vi "Handle LogRec.vi"(8 "error in":errorcluster, 10 "LogRecord":refnum<class "LogRecord.lvclass">, 11 "LokiHandler in":refnum<class "LokiHandler.lvclass">) -> (0 "error out":errorcluster, 3 "LokiHandler out":refnum<class "LokiHandler.lvclass">)   [LabVIEW 2017, in "hse-logger.lvlib" / "LokiHandler.lvclass"]
doc: "Handles the incoming ``LogRecord`` object.\n\nThis method is the implementation of the base-class and does nothing. Use a pre-defined sub-class or implement your own."
uses:
  LokiHandler.lvclass
  LokiHandler.lvclass/LokiHandler.ctl
  LogRecord/LogRecord.lvclass
  <vilib>/httpClient/LabVIEWHTTPClient.lvlib
  <vilib>/httpClient/POSTBuffer.vi
  Formatter/LokiJsonFormatter/LokiJsonFormatter.lvclass
panel:
  # "Connector Pane"
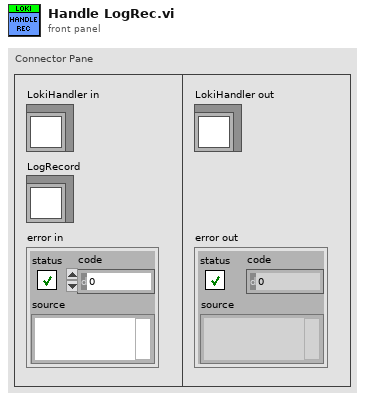
[diagram p1: front panel]
types:
  T1 = typedef "hse-logger.lvlib/LogLevel.ctl" = enum16{"DEBUG", "INFO", "WARNING", "ERROR", "CRITICAL"}
  T2 = typedef "LabVIEWHTTPClient.lvlib/ClientHandle.ctl" = refnum<k1>
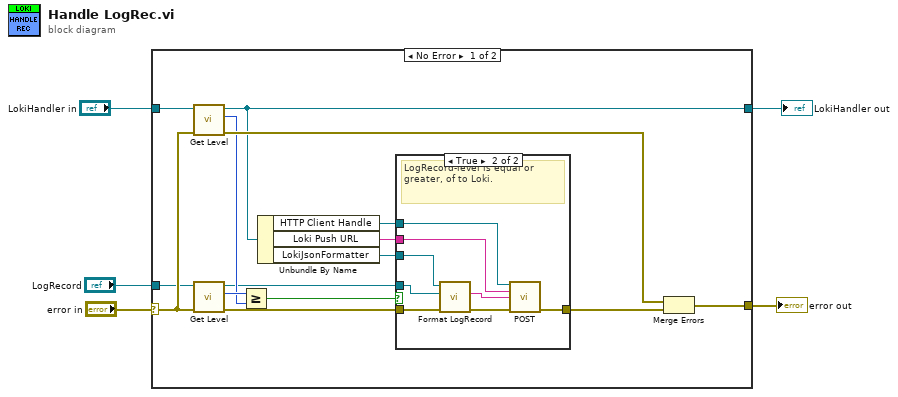
[diagram p0: block diagram]
diagram:
  n1 = case shown="No Error" "error in" {
    selector: "error in" -> [w19 w31]
    tunnel: [w10 w31] -> w1
    tunnel: [w12 w30] -> w2
    tunnel: "LokiHandler in" -> [w18 w30]
    tunnel: "LogRecord" -> [w17 _]
    frame No Error {
      n2 = call-dynamic "Get Level.vi"("error in"=w19, "Handler in"=w18) -> ("error out"=w20:errorcluster, "Level"=w15:T1, "Handler out"=w12:refnum<class "LokiHandler.lvclass">)  [unwired: 7 in]
      n3 = call "Get Level.vi"("error in"=w19, "LogRecord in"=w17) -> ("error out"=w13:errorcluster, "Level"=w16:T1, "LogRecord out"=w11:refnum<class "LogRecord.lvclass">)  [unwired: 7 in]
      n4 = Greater Or Equal?(x=w16, y=w15) -> (x >= y?=w14:bool)
      n5 = Unbundle By Name(w12) -> ("HTTP Client Handle"=w8:T2, "Loki Push URL"=w7:string, "LokiJsonFormatter"=w6:refnum<class "LokiJsonFormatter.lvclass">)
      n6 = case shown="True" w14 {
        tunnel: w13 -> [w21 w28]
        tunnel: w11 -> [_ w26]
        tunnel: [w21 w29] -> w9
        tunnel: w8 -> [_ w25]
        tunnel: w7 -> [_ w24]
        tunnel: w6 -> [_ w22]
        frame False {
          # "Do not write to file."
        }
        frame True {
          # "LogRecord-level is equal or greater, of to Loki."
          n7 = call-dynamic "Format LogRecord.vi"("error in"=w28, "LogRecord"=w26, "LokiJsonFormatter in"=w22) -> ("error out"=w27:errorcluster, "LogLine"=w23:string)  [unwired: 7 in]
          n8 = call-poly <vilib>:"POST.vi"("client handle"=w25, "url"=w24, "buffer"=w23, "error in (no error)"=w27) -> ("error out"=w29:errorcluster)  [unwired: 8 in, 3 out]
        }
      }
      n9 = Merge Errors(w20, w9) -> (w10:errorcluster)
    }
    frame Error {
    }
  }
  "error out" <- w1
  "LokiHandler out" <- w2
